vi "sequencerCore.vi"   [LabVIEW 2014]
uses:
  sequencerState.ctl
  <vilib>/rvi/Emulation/niFpgaGetClockAttributes.vi
  <vilib>/rvi/Emulation/niFpgaSctlEmulationGetInTimedLoop.vi
  <vilib>/rvi/Emulation/niFpgaEmulationReportErrorSimple.vi
  DAC/Code/FPGA SPI_Globals.vi
  <vilib>/rvi/Emulation/niFpgaCriticalErrorInLSC.vi
types:
  T1 = typedef "sequencerState.ctl" = enum16{"init", "idle", "measureOffset", "measureTrack", "measComplete", "error"}
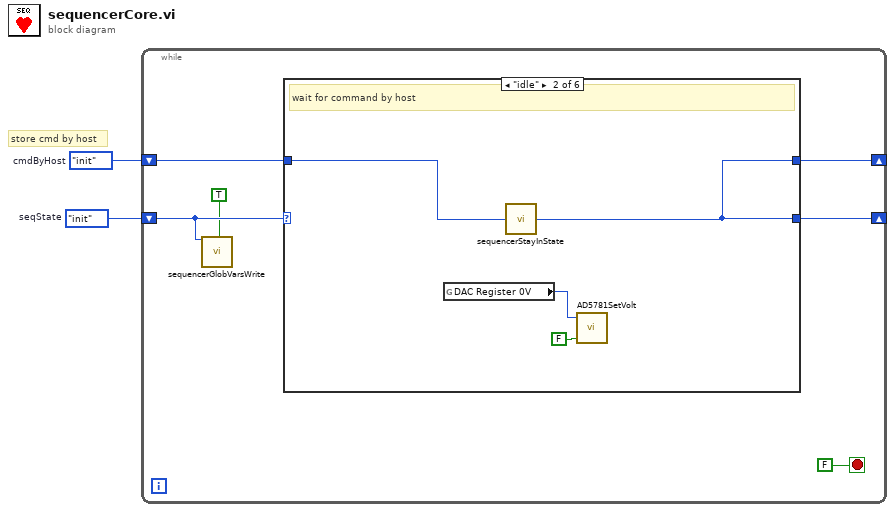
[diagram p0: block diagram]
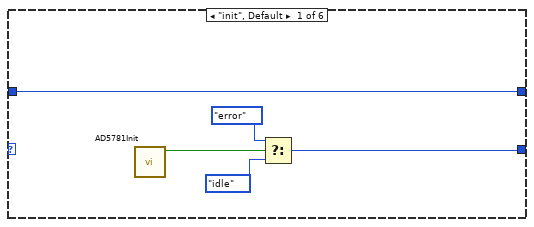
[diagram p2: hidden frame]
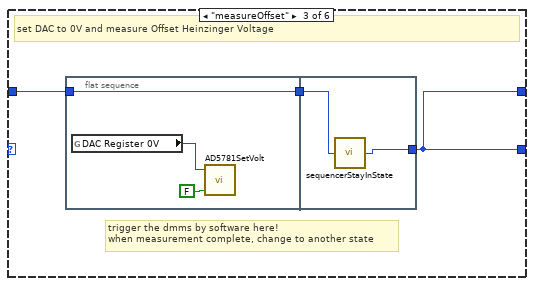
[diagram p3: hidden frame]
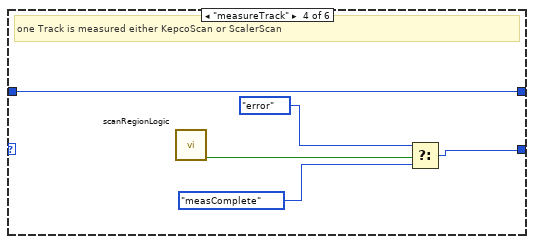
[diagram p4: hidden frame]
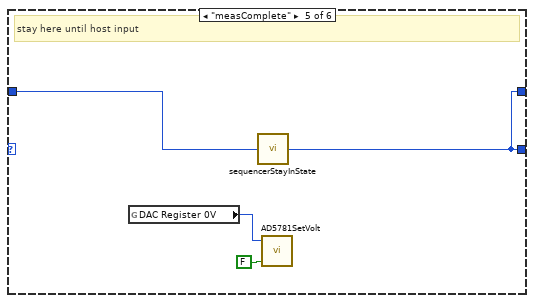
[diagram p5: hidden frame]
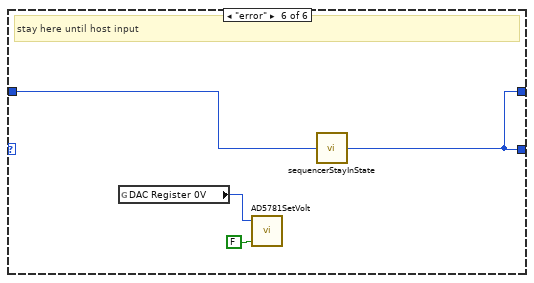
[diagram p6: hidden frame]
diagram:
  w1 = sequencerState."init"  # cmdByHost
  w2 = sequencerState."init"  # seqState
  # "store cmd by host"
  n1 = while {
    shift-right: [w6] -> _
    shift-left: w2 -> [w7]
    shift-right: [w4] -> _
    shift-left: w1 -> [w3]
    stop <- FALSE stop-if-true
    n2 = call "sequencerGlobVarsWrite.vi"("seqState"=w7, "writeOnlySeqState"=TRUE ("seqStateWired?")) -> ()  [unwired: 18 in]
    n3 = case shown="\"idle\"" w7 {
      tunnel: [w10 w17 w19 w27 w33 w37] -> w6
      tunnel: [w9 w17 w19 w26 w33 w37] -> w4
      tunnel: w3 -> [w9 w16 w20 w26 w34 w38]
      frame "init", Default {
        n4 = call "AD5781Init.vi"() -> ("timeOut"=w11:bool)  [unwired: 11 in]
        n5 = Select(t=sequencerState."error", s=w11, f=sequencerState."idle" ("Enum")) -> (s? t:f=w10:T1)
      }
      frame "idle" {
        # "wait for command by host"
        n6 = global read "FPGA SPI_Globals.vi" "DAC Register 0V"() -> (w14:u32)
        n7 = call "sequencerStayInState.vi"("stateBefore"=w16) -> ("cmdByHost"=w17:T1)  [unwired: 4 in]
        n8 = call "AD5781SetVolt.vi"("Send"=FALSE, "SetVolt"=w14) -> ()  [unwired: 1 in, 3 out]
      }
      frame "measureOffset" {
        # "trigger the dmms by software here!\nwhen measurement complete, change to another state"
        # "set DAC to 0V and measure Offset Heinzinger Voltage"
        n9 = flat-sequence {
          tunnel: w20 -> [w23]
          tunnel: [w23] -> w18
          tunnel: [w24] -> w19
          tunnel: w18 -> [w25]
          frame #0 {
            n10 = global read "FPGA SPI_Globals.vi" "DAC Register 0V"() -> (w21:u32)
            n11 = call "AD5781SetVolt.vi"("Send"=FALSE, "SetVolt"=w21) -> ()  [unwired: 1 in, 3 out]
          }
          frame #1 {
            n12 = call "sequencerStayInState.vi"("stateBefore"=w25) -> ("cmdByHost"=w24:T1)  [unwired: 4 in]
          }
        }
      }
      frame "measureTrack" {
        # "one Track is measured either KepcoScan or ScalerScan"
        n13 = call "scanRegionLogic.vi"() -> ("Error"=w28:bool)  [unwired: 11 in]
        n14 = Select(t=sequencerState."error" ("Enum"), s=w28, f=sequencerState."measComplete" ("Enum")) -> (s? t:f=w27:T1)
      }
      frame "measComplete" {
        # "stay here until host input"
        n15 = global read "FPGA SPI_Globals.vi" "DAC Register 0V"() -> (w31:u32)
        n16 = call "sequencerStayInState.vi"("stateBefore"=w34) -> ("cmdByHost"=w33:T1)  [unwired: 4 in]
        n17 = call "AD5781SetVolt.vi"("Send"=FALSE, "SetVolt"=w31) -> ()  [unwired: 1 in, 3 out]
      }
      frame "error" {
        # "stay here until host input"
        n18 = global read "FPGA SPI_Globals.vi" "DAC Register 0V"() -> (w35:u32)
        n19 = call "AD5781SetVolt.vi"("Send"=FALSE, "SetVolt"=w35) -> ()  [unwired: 1 in, 3 out]
        n20 = call "sequencerStayInState.vi"("stateBefore"=w38) -> ("cmdByHost"=w37:T1)  [unwired: 4 in]
      }
    }
  }
